vi "SVT Audio Filter (N Ch).vi"(6 "reset filter (F)":bool, 8 "error in (no error)":errorcluster, 10 "filter type":u16(ring) items=["Linear"=0, "AES17 20 kHz Lowpass"=17, "AES17 40 kHz Lowpass"=18, "AES17 20 kHz Highpass"=19, "AES17 40 kHz Highpass"=20], 11 "scaled signals [EU]":waveform(dbl)[](array[waveform])) -> (0 "error out":errorcluster, 1 "phase response":cluster{"f0":dbl, "df":dbl, "Phase":dbl[]}, 2 "magnitude response":cluster{"f0":dbl, "df":dbl, "Mag":dbl[]}, 3 "filtered signals [EU]":waveform(dbl)[](array[waveform]))   [LabVIEW 2017, in "SoundVib_AudioFilter.lvlib"]
doc: "Applies the selected audio weighting filter to the <B>scaled signal [EU]</B>. Wire data to the <B>scaled signal [EU]</B> input to determine the polymorphic instance to use or manually select the instance."
uses:
  <vilib>/addons/Sound and Vibration/svt_Weighting/SoundVib_AudioFilter.lvlib
  <vilib>/addons/_NISVFA/_Shared subVIs/Common/svc_Check for Waveform Parameter Continuity (no state).vi
  <vilib>/addons/_NISVFA/_Shared subVIs/Common/svc_Get SV Channel Info.vi
  <vilib>/addons/_NISVFA/_Shared subVIs/Common/svc_Engineering Units to Unit Label.vi
  <vilib>/addons/_NISVFA/_Shared subVIs/Common/svc_Unit Label to Engineering Units.vi
  <vilib>/Analysis/NI_AALBase.lvlib
  <vilib>/measure/NI_MAPro.lvlib
  <vilib>/measure/NI_MABase.lvlib
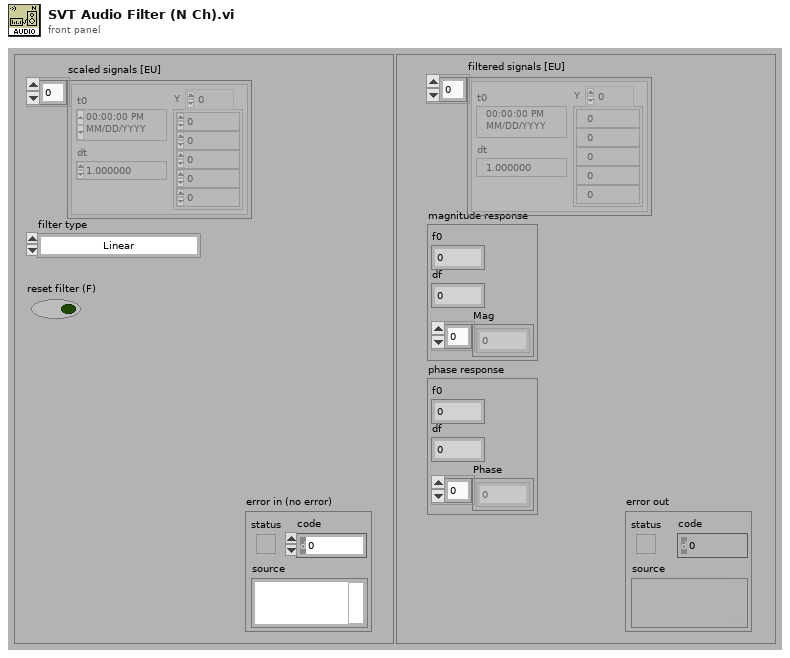
[diagram p1: front panel]
types:
  T1 = cluster{"dt equal":bool, "array length equal":bool, "number channels change":bool}
  T2 = cluster{"dt":bool, "t0 continuity":bool, "array length":bool, "channel info":bool, "name":bool}
  T3 = enum32{"Lowpass", "Highpass", "Bandpass", "Bandstop"}
  T4 = typedef "svc_Weighting Filter Text Ring.ctl" = u16
  T5 = cluster{"filter structure":enum32{"IIR 2nd Order", "IIR 4th Order"}, "Reverse Coefficients":dbl[], "Forward Coefficients":dbl[]}
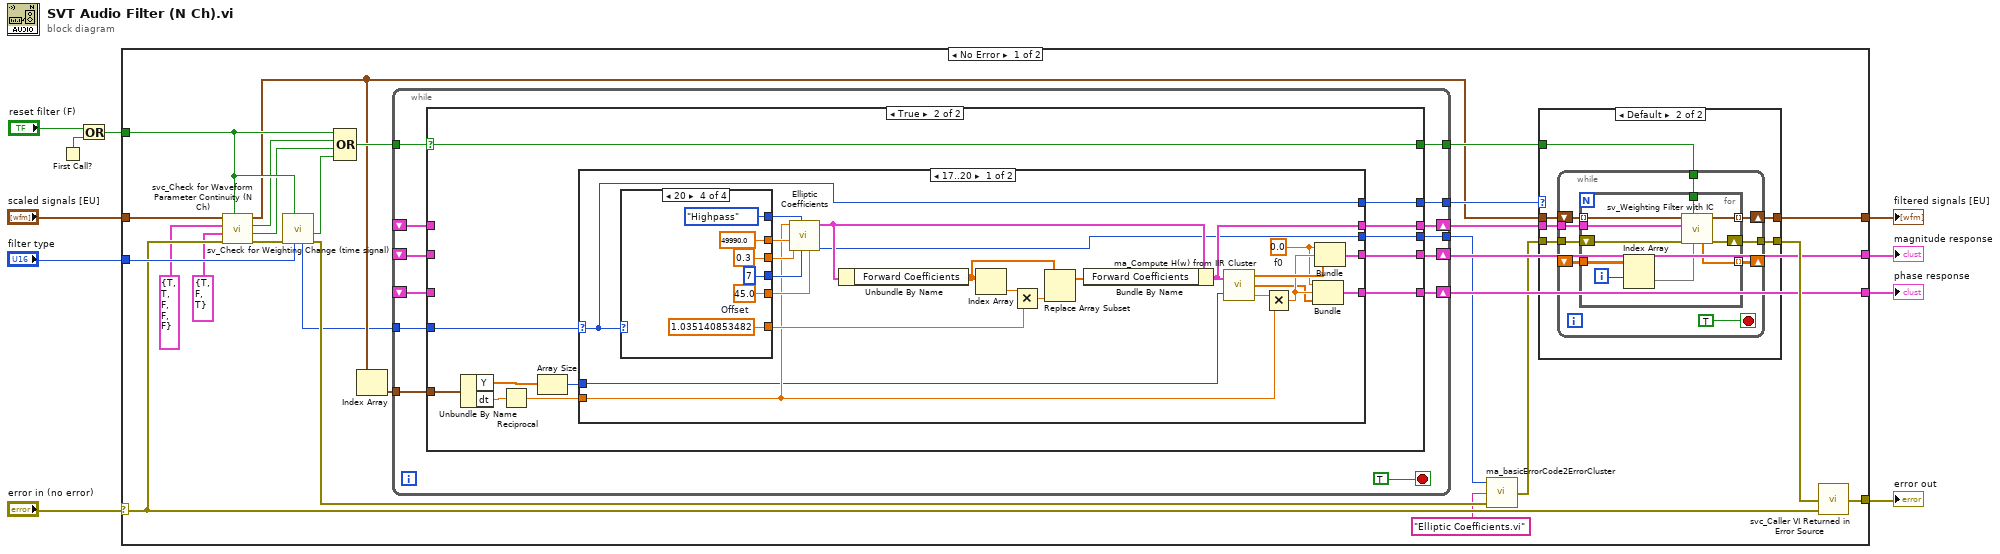
[diagram p0: block diagram]
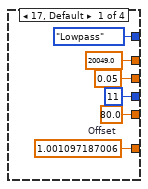
[diagram p4: hidden frame]
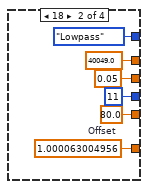
[diagram p5: hidden frame]
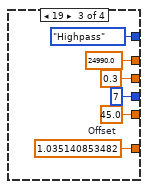
[diagram p6: hidden frame]
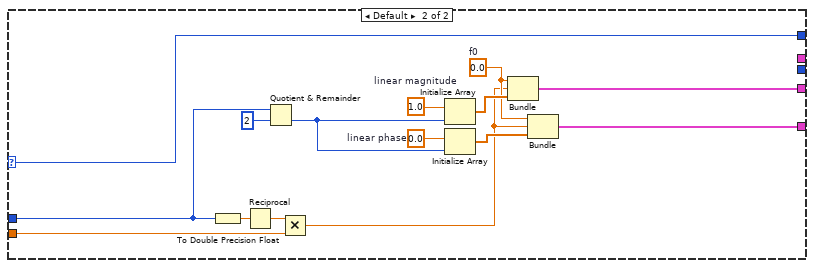
[diagram p7: hidden frame]
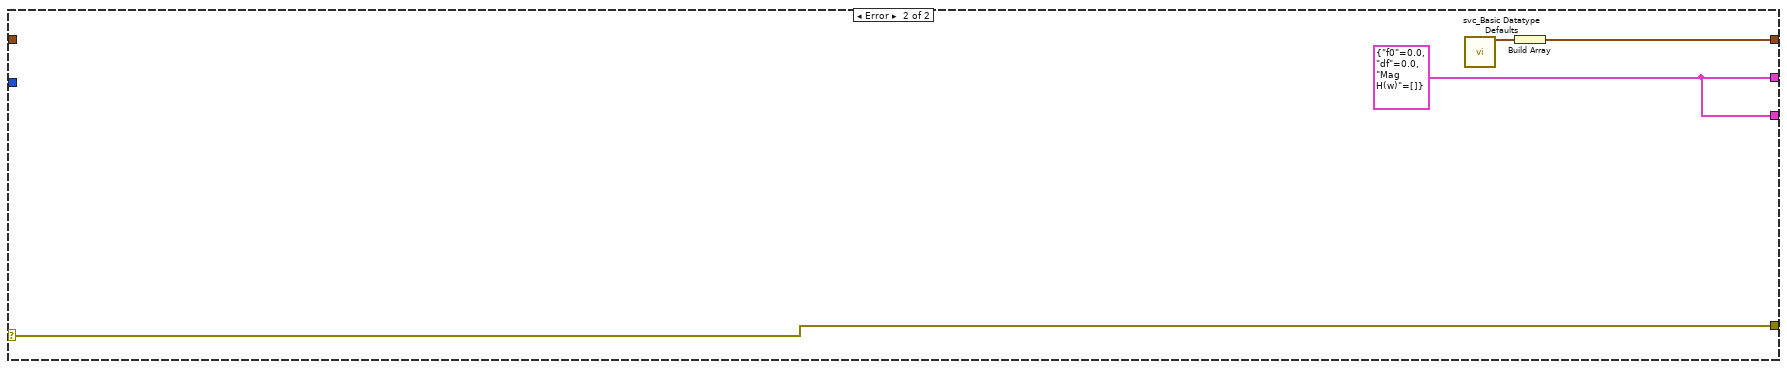
[diagram p8: hidden frame]
diagram:
  n1 = First Call?() -> (First Call?: T/F=w5:bool)
  n2 = Or(x="reset filter (F)", y=w5) -> (x .or. y?=w9:bool)
  n3 = case shown="No Error" "error in (no error)" {
    selector: "error in (no error)" -> [w25 w159]
    tunnel: [w35 w159] -> w10
    tunnel: [w32 w157] -> w3
    tunnel: "scaled signals [EU]" -> [w27 _]
    tunnel: w9 -> [w23 _]
    tunnel: "filter type" -> [w28 _]
    tunnel: [w34 w156] -> w1
    tunnel: [w33 w156] -> w2
    frame No Error {
      n4 = call <vilib>:"svc_Check for Waveform Parameter Continuity (N Ch).vi"("restart averaging (F)"=w23, "error in (no error)"=w25, "checks for multichannel parameters"=T1 {"dt equal"=TRUE, "array length equal"=FALSE, "number channels change"=TRUE}, "checks for channel parameter change"=T2 {"dt"=TRUE, "t0 continuity"=TRUE, "array length"=FALSE, "channel info"=FALSE, "name"=FALSE}, "scaled signal(s)"=w27) -> ("error out"=w26:errorcluster, "multichannel parameter changed"=w21:bool, "waveform parameter changed"=w22:bool, "dup scaled signal(s)"=w19:waveform(dbl)[])  [unwired: 3 out]
      n5 = call <vilib>:"sv_Check for Weighting Change (time signal).vi"("weighting"=w28, "reset (in)"=w23, "error in (no error)"=w26) -> ("error out"=w16:errorcluster, "weighting has changed"=w20:bool, "dup weighting"=w13:T4)  [unwired: 6 in]
      n6 = Compound Arithmetic op=OR(w23, w22, w21, w20) -> (w24:bool)
      n7 = Index Array(array=w19) -> (element=w18:waveform(dbl))  [unwired: 1 in]
      n8 = while {
        shift-right: [w75] -> w29
        shift-left: _ -> [w76]
        shift-right: [w74] -> w33
        shift-left: _ -> [w71]
        shift-right: [w73] -> w34
        shift-left: _ -> [w72]
        tunnel: [w70] -> w30
        tunnel: w13 -> [w69]
        tunnel: [w68] -> w31
        tunnel: w24 -> [w67]
        tunnel: w18 -> [w66]
        tunnel: [w64] -> w17
        stop <- TRUE stop-if-true
        n9 = case shown="True" w67 {
          selector: w67 -> [w78 w89]
          tunnel: w66 -> [_ w93]
          tunnel: w76 -> [w81 _]
          tunnel: [w81 w92] -> w75
          tunnel: [w80 w91] -> w74
          tunnel: [w79 w90] -> w73
          tunnel: w72 -> [w79 _]
          tunnel: w71 -> [w80 _]
          tunnel: [w78 w89] -> w70
          tunnel: w69 -> [w77 w87]
          tunnel: [w77 w88] -> w68
          tunnel: [_ w82] -> w64
          frame False {
            # "Filter is not reset"
          }
          frame True {
            n10 = Unbundle By Name(w93) -> ("Y"=w84:dbl[], "dt"=w86:dbl)
            n11 = Reciprocal(x=w86) -> (1/x=w85:dbl)
            n12 = Array Size(array=w84) -> (size(s)=w83:i32)
            n13 = case shown="17..20" w87 {
              selector: w87 -> [w103 w149]
              tunnel: w85 -> [w96 w147]
              tunnel: [w110 _] -> w92
              tunnel: [w108 w150] -> w91
              tunnel: [w104 w151] -> w90
              tunnel: [w103 w149] -> w88
              tunnel: w83 -> [w95 w141]
              tunnel: [w94 _] -> w82
              frame 17..20 {
                w105 = 0.0  # f0
                n14 = case shown="20" w103 {
                  tunnel: [w122 w128 w134 w140] -> w115
                  tunnel: [T3."Lowpass" ("filter type") T3."Lowpass" ("filter type") T3."Highpass" ("filter type") T3."Highpass" ("filter type")] -> w102
                  tunnel: [20049.0 ("low cutoff freq: fl") 40049.0 ("low cutoff freq: fl") 24990.0 ("low cutoff freq: fl") 49990.0 ("low cutoff freq: fl")] -> w98
                  tunnel: [11 ("order") 11 ("order") 7 ("order") 7 ("order")] -> w100
                  tunnel: [80.0 ("stopband attenuation (dB)") 80.0 ("stopband attenuation (dB)") 45.0 ("stopband attenuation (dB)") 45.0 ("stopband attenuation (dB)")] -> w99
                  tunnel: [0.05 ("low cutoff freq: fl") 0.05 ("low cutoff freq: fl") 0.3 ("low cutoff freq: fl") 0.3 ("low cutoff freq: fl")] -> w97
                  frame 17, Default {
                    w122 = 1.001097187006  # Offset
                  }
                  frame 18 {
                    w128 = 1.000063004956  # Offset
                  }
                  frame 19 {
                    w134 = 1.035140853482  # Offset
                  }
                  frame 20 {
                    w140 = 1.035140853482  # Offset
                  }
                }
                n15 = call <vilib>:"Elliptic Coefficients.vi"("stopband attenuation (dB)"=w99, "order"=w100, "filter type"=w102, "passband ripple (dB)"=w97, "low cutoff freq: fl"=w98, "sampling freq: fs"=w96) -> ("error"=w94:i32, "IIR Filter Cluster"=w101:T5)  [unwired: 4 in]
                n16 = Unbundle By Name(w101) -> ("Forward Coefficients"=w114:dbl[])
                n17 = Index Array(array=w114) -> (element=w116:dbl)  [unwired: 1 in]
                n18 = Multiply(x=w116, y=w115) -> (x*y=w113:dbl)
                n19 = Replace Array Subset(array=w114, new element=w113) -> (w112:dbl[])  [unwired: 1 in]
                n20 = Bundle By Name(cluster=w101, "Forward Coefficients"=w112) -> (w110:T5)
                n21 = call <vilib>:"ma_Compute H(w) from IIR Cluster.vi"("IIR Filter Cluster"=w110, "FFT size"=w95) -> ("Mag H(w)"=w109:dbl[], "Phase H(w)"=w106:dbl[], "df"=w111:dbl)
                n22 = Multiply(x=w111, y=w96) -> (x*y=w107:dbl)
                n23 = Bundle("f0"=w105, w107, "Phase H(w)"=w106) -> (w104:cluster{"f0":dbl, dbl, "Phase H(w)":dbl[]})  [unwired: 1 in]
                n24 = Bundle("f0"=w105, w107, "Mag H(w)"=w109) -> (w108:cluster{"f0":dbl, dbl, "Mag H(w)":dbl[]})  [unwired: 1 in]
              }
              frame Default {
                w155 = 1.0  # linear magnitude
                w153 = 0.0  # linear phase
                w146 = 0.0  # f0
                n25 = To Double Precision Float(number=w141) -> (double precision float=w144:dbl)
                n26 = Reciprocal(x=w144) -> (1/x=w148:dbl)
                n27 = Quotient & Remainder(x=w141, y=2) -> (floor(x/y)=w142:i32)  [unwired: 1 out]
                n28 = Multiply(x=w148, y=w147) -> (x*y=w145:dbl)
                n29 = Initialize Array(w155, w142) -> (w152:dbl[])
                n30 = Initialize Array(w153, w142) -> (w154:dbl[])
                n31 = Bundle("f0"=w146, w145, w152) -> (w150:cluster{"f0":dbl, dbl, dbl[]})  [unwired: 1 in]
                n32 = Bundle("f0"=w146, w145, w154) -> (w151:cluster{"f0":dbl, dbl, dbl[]})  [unwired: 1 in]
              }
            }
          }
        }
      }
      n33 = call <vilib>:"ma_basicErrorCode2ErrorCluster.vi"("error in (no error)"=w16, "subVI name"="Elliptic Coefficients.vi", "Error Code"=w17) -> ("error out"=w15:errorcluster)
      n34 = case shown="Default" w31 {
        tunnel: [w38 w39] -> w32
        tunnel: w29 -> [_ w44]
        tunnel: w30 -> [_ w43]
        tunnel: w19 -> [w38 w40]
        tunnel: w15 -> [w37 w42]
        tunnel: [w37 w41] -> w36
        frame 0 {
        }
        frame Default {
          n35 = while {
            tunnel: w44 -> [w53]
            tunnel: w43 -> [w52]
            tunnel: w42 -> [w51]
            tunnel: [w50] -> w41
            shift-right: [w48] -> w39
            shift-left: w40 -> [w49]
            shift-right: [w47] -> _
            shift-left: _ -> [w46]
            stop <- TRUE stop-if-true
            n36 = for {
              tunnel: [w63] -> w48 mode=indexing
              tunnel: w53 -> [w62]
              tunnel: w52 -> [w61]
              tunnel: w49 -> [w60] mode=indexing
              shift-right: [w58] -> w50
              shift-left: w51 -> [w59]
              tunnel: [w56] -> w47 mode=indexing
              tunnel: w46 -> [w55]
              i -> [w57]
              n37 = Index Array(array=w55, index (row)=w57) -> (element=w54:dbl[])  [unwired: 1 in]
              n38 = call <vilib>:"sv_Weighting Filter with IC.vi"("Initial Filter State"=w54, "error in (no error)"=w59, "reset filter (F)"=w61, "filter coefficients"=w62, "signal [V]"=w60) -> ("error out"=w58:errorcluster, "filtered signal [EU]"=w63:waveform(dbl), "Final Filter State"=w56:dbl[])  [unwired: 4 in]
            }
          }
        }
      }
      n39 = call <vilib>:"svc_Caller VI Returned in Error Source.vi"("warning input to caller"=w25, "error in (no error)"=w36) -> ("error out"=w35:errorcluster)  [unwired: 3 in]
    }
    frame Error {
      w156 = cluster{"f0":dbl, "df":dbl, "Mag H(w)":dbl[]} {"f0"=0.0, "df"=0.0, "Mag H(w)"=[]} ("magnitude H(w)")
      n40 = call <vilib>:"svc_Basic Datatype Defaults.vi"() -> ("empty waveform"=w158:waveform(dbl))  [unwired: 7 in, 12 out]
      n41 = Build Array(w158) -> (w157:waveform(dbl)[])
    }
  }
  "error out" <- w10
  "magnitude response" <- w2
  "phase response" <- w1
  "filtered signals [EU]" <- w3
